vi "Test Instrument Manager Virtual NEO480 cRIO XNET.vi"(11 "Test Case In":refnum<class "Test Instrument Manager.lvclass">) -> (0 "error out":errorcluster, 3 "Test Case Out":refnum<class "Test Instrument Manager.lvclass">)   [LabVIEW 2024, in "Test Instrument Manager.lvclass"]
uses:
  Test Instrument Manager.lvclass
  C:/Program Files/National Instruments/LabVIEW 2025/vi.lib/Astemes/LUnit/Test Case.lvclass
  Source/Virtual NEO480/Virtual NEO480.lvclass
  Source/Config from JSON/Config from JSON.lvclass
  D:/git/HAL/Source/Interfaces/IConfiguration/IConfiguration.lvclass
  <vilib>/Astemes/LUnit/Test Case.lvclass/Test Case.ctl
  Test Instrument Manager.lvclass/Test Instrument Manager.ctl
  <vilib>/Astemes/LUnit/Test Case.lvclass
  Source/Instrument Manager/Instrument Manager.lvclass
panel:
  out "Temperature":dbl
  out "Time Stamp":timestamp format="%<%x %.3X>T"
  in  "stop":bool
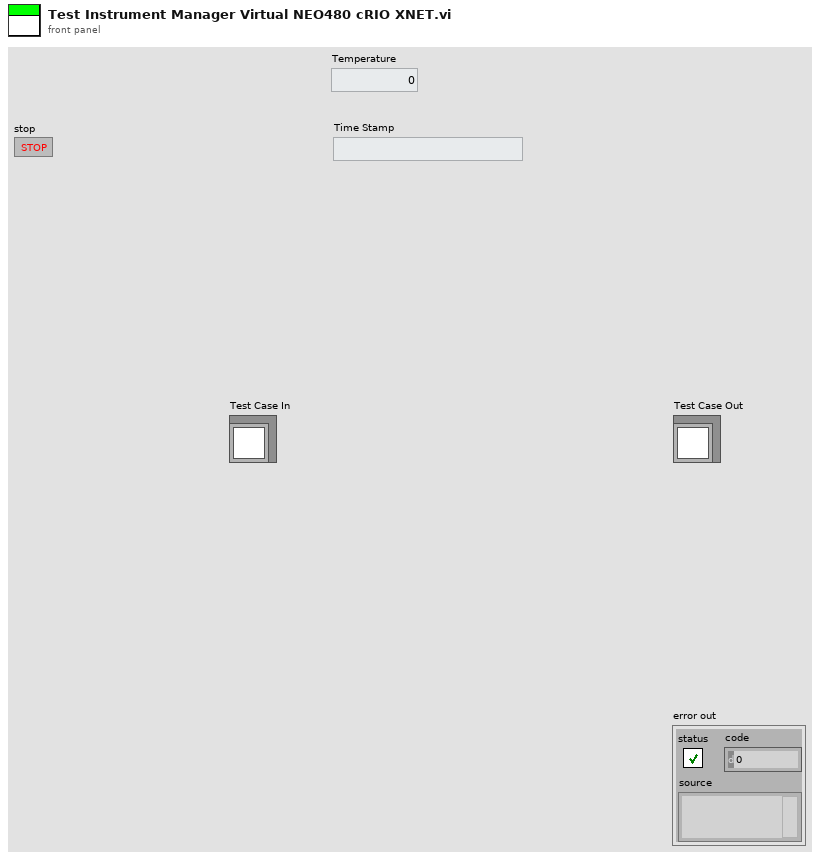
[diagram p1: front panel]
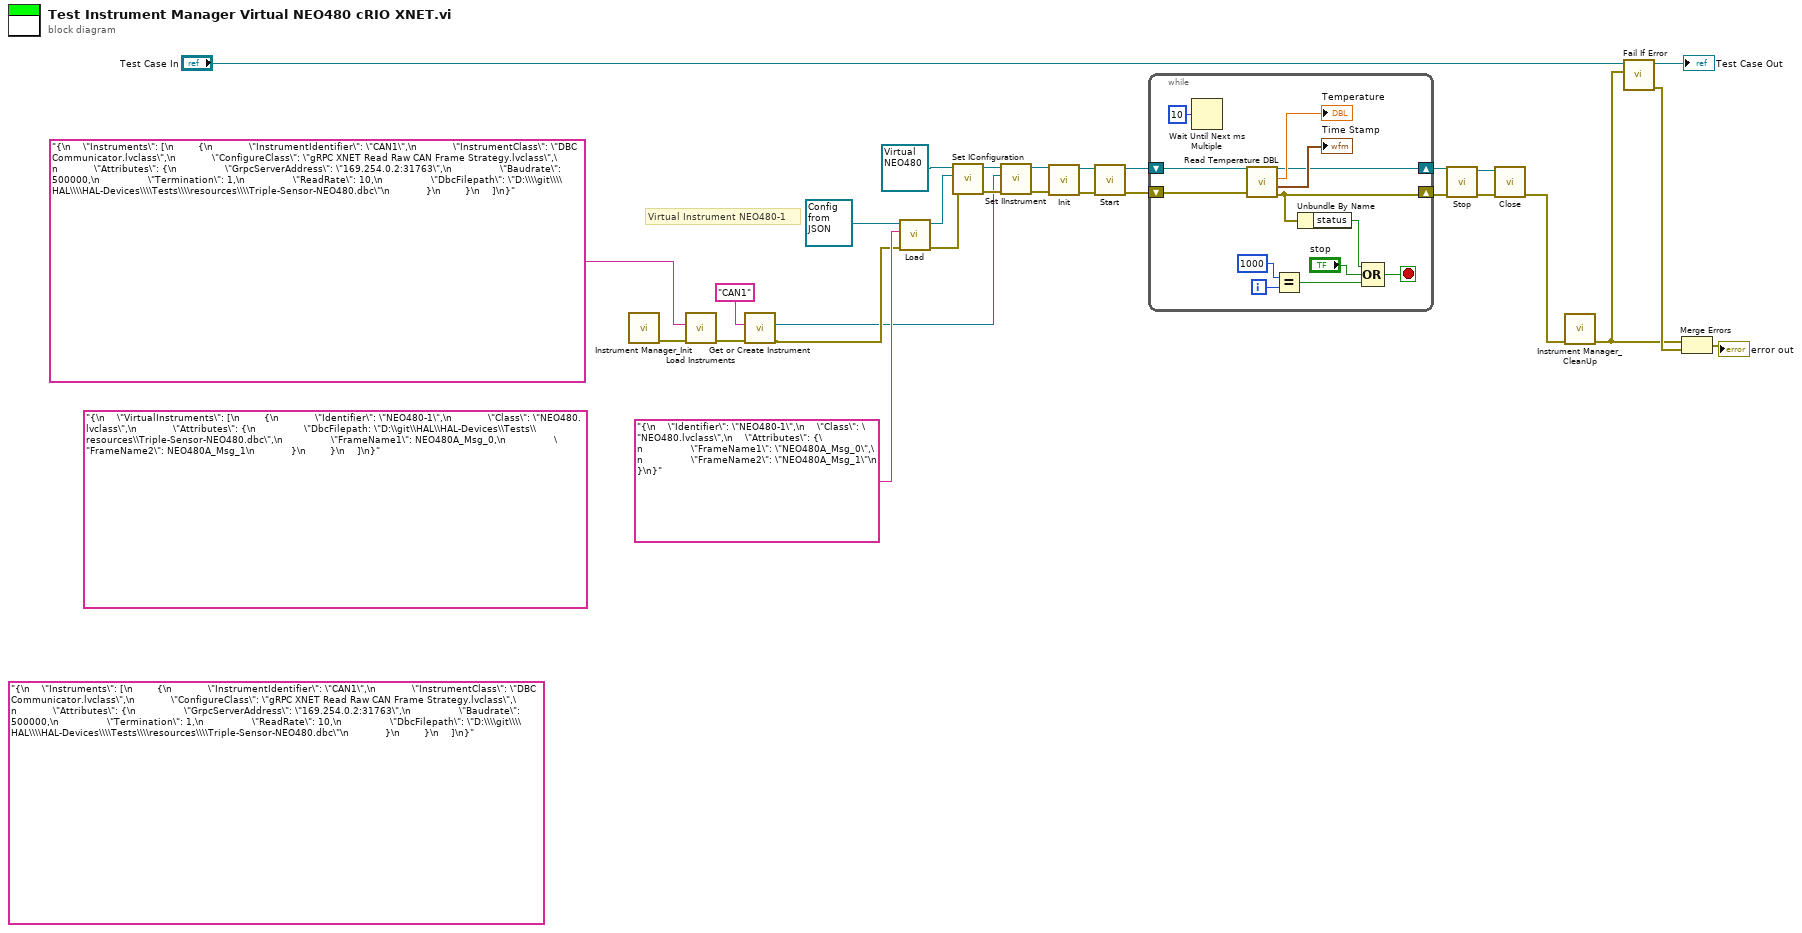
[diagram p0: block diagram]
diagram:
  (unwired) "{\n    \"VirtualInstruments\": [\n        {\n            \"Identifier\": \"NEO480-1\",\n            \"Class\": \"NEO480.lvclass\",\n            \"Attributes\": {\n                \"DbcFilepath: \"D:\\git\\HAL\\HAL-Devices\\Tests\\resources\\Triple-Sensor-NEO480.dbc\",\n                \"FrameName1\": NEO480A_Msg_0,\n                \"FrameName2\": NEO480A_Msg_1\n            }\n        }\n    ]\n}"
  (unwired) "{\n    \"Instruments\": [\n        {\n            \"InstrumentIdentifier\": \"CAN1\",\n            \"InstrumentClass\": \"DBC Communicator.lvclass\",\n            \"ConfigureClass\": \"gRPC XNET Read Raw CAN Frame Strategy.lvclass\",\n            \"Attributes\": {\n                \"GrpcServerAddress\": \"169.254.0.2:31763\",\n                \"Baudrate\": 500000,\n                \"Termination\": 1,\n                \"ReadRate\": 10,\n                \"DbcFilepath\": \"D:\\\\git\\\\HAL\\\\HAL-Devices\\\\Tests\\\\resources\\\\Triple-Sensor-NEO480.dbc\"\n            }\n        }\n    ]\n}" ("Source")
  # "Virtual Instrument NEO480-1"
  n1 = call "Instrument Manager_Init.vi"() -> ("Error Out"=w7:errorcluster)  [unwired: 10 in, 1 out]
  n2 = call "Load Instruments.vi"("Error In"=w7, "Source"="{\n    \"Instruments\": [\n        {\n            \"InstrumentIdentifier\": \"CAN1\",\n            \"InstrumentClass\": \"DBC Communicator.lvclass\",\n            \"ConfigureClass\": \"gRPC XNET Read Raw CAN Frame Strategy.lvclass\",\n            \"Attributes\": {\n                \"GrpcServerAddress\": \"169.254.0.2:31763\",\n                \"Baudrate\": 500000,\n                \"Termination\": 1,\n                \"ReadRate\": 10,\n                \"DbcFilepath\": \"D:\\\\git\\\\HAL\\\\HAL-Devices\\\\Tests\\\\resources\\\\Triple-Sensor-NEO480.dbc\"\n            }\n        }\n    ]\n}") -> ("Error Out"=w6:errorcluster)  [unwired: 9 in]
  n3 = call "Get or Create Instrument.vi"("Error In"=w6, "Instrument Identifier"="CAN1") -> ("Error Out"=w5:errorcluster, "IInstrument"=w3:refnum<class "IInstrument.lvclass">)  [unwired: 8 in]
  n4 = call-dynamic "Load.vi"("error in"=w5, "Source"="{\n    \"Identifier\": \"NEO480-1\",\n    \"Class\": \"NEO480.lvclass\",\n    \"Attributes\": {\n                \"FrameName1\": \"NEO480A_Msg_0\",\n                \"FrameName2\": \"NEO480A_Msg_1\"\n    }\n}", "Config From JSON in"=refnum<class "Config from JSON.lvclass"> refnum ("Config from JSON.lvclass")) -> ("error out"=w10:errorcluster, "Config From JSON out"=w23:refnum<class "Config from JSON.lvclass">)  [unwired: 7 in]
  n5 = call-dynamic "Set IConfiguration.vi"("IConfiguration"=w23, "NEO480 in"=refnum<class "Virtual NEO480.lvclass"> refnum ("NEO480.lvclass")) -> ("NEO480 out"=w22:refnum<class "Virtual NEO480.lvclass">)  [unwired: 9 in]
  n6 = call-dynamic "Set IInstrument.vi"("error in"=w10, "IInstrument"=w3, "NEO480 in"=w22) -> ("error out"=w11:errorcluster, "NEO480 out"=w19:refnum<class "Virtual NEO480.lvclass">)  [unwired: 7 in]
  n7 = call-dynamic "Init.vi"("error in"=w11, "NEO480 in"=w19) -> ("error out"=w14:errorcluster, "NEO480 out"=w21:refnum<class "Virtual NEO480.lvclass">)  [unwired: 8 in]
  n8 = call-dynamic "Start.vi"("error in"=w14, "NEO480 in"=w21) -> ("error out"=w13:errorcluster, "NEO480 out"=w20:refnum<class "Virtual NEO480.lvclass">)  [unwired: 8 in]
  n9 = while {
    shift-right: [w30] -> w17
    shift-left: w20 -> [w39]
    shift-right: [w31] -> w18
    shift-left: w13 -> [w29]
    i -> [w36]
    stop <- w37 stop-if-true
    n10 = Wait Until Next ms Multiple(millisecond multiple=u32 10) -> ()  [unwired: 1 out]
    n11 = call-dynamic "Read Temperature DBL.vi"("error in"=w29, "NEO480 in"=w39) -> ("error out"=w31:errorcluster, "Time Stamp"=→"Time Stamp":timestamp, "Temperature"=→"Temperature":dbl, "NEO480 out"=w30:refnum<class "Virtual NEO480.lvclass">)  [unwired: 6 in]
    n12 = Equal?(x=1000, y=w36) -> (x = y?=w33:bool)
    n13 = Unbundle By Name(w31) -> ("status"=w32:bool)
    n14 = Compound Arithmetic op=OR(w32, "stop", w33) -> (w37:bool)
  }
  n15 = call-dynamic "Stop.vi"("error in"=w18, "NEO480 in"=w17) -> ("error out"=w16:errorcluster, "NEO480 out"=w15:refnum<class "Virtual NEO480.lvclass">)  [unwired: 8 in]
  n16 = call-dynamic "Close.vi"("error in"=w16, "NEO480 in"=w15) -> ("error out"=w2:errorcluster)  [unwired: 8 in, 1 out]
  n17 = call "Instrument Manager_CleanUp.vi"("Error In"=w2) -> ("Error Out"=w1:errorcluster)  [unwired: 10 in]
  n18 = call <vilib>:"Fail If Error.vi"("Assert error"=w1, "LUnit Test Case In"="Test Case In") -> ("error out"=w26:errorcluster, "LUnit Test Case Out"=→"Test Case Out":refnum<class "Test Instrument Manager.lvclass">)  [unwired: 8 in]
  n19 = Merge Errors(w1, w26) -> (→"error out":errorcluster)
